vi "write error in txt.vi"(8 "error in (no error)":errorcluster caption="错误输入（无错误）", 9 "file name":string, 11 "path":path) -> (0 "error out":errorcluster, 3 "path":path)   [LabVIEW 2018]
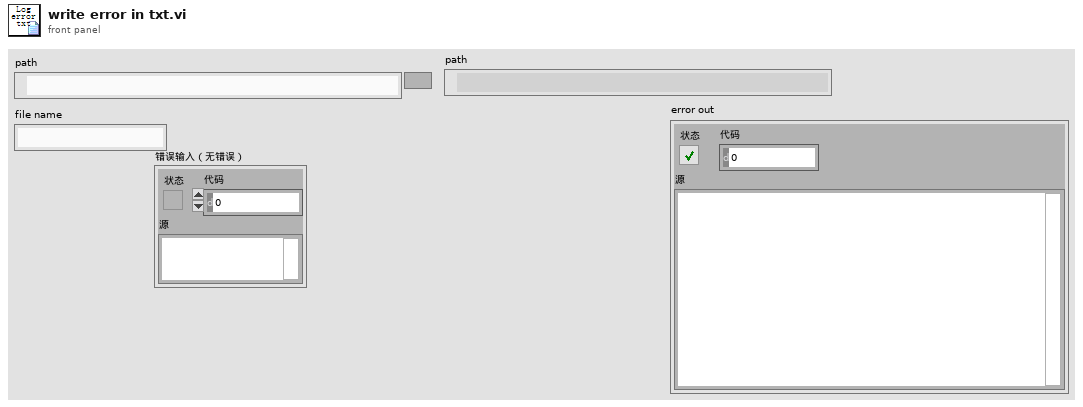
[diagram p1: front panel]
types:
  T1 = enum16{"open", "replace", "create", "open or create", "replace or create", "replace or create with confirmation"}
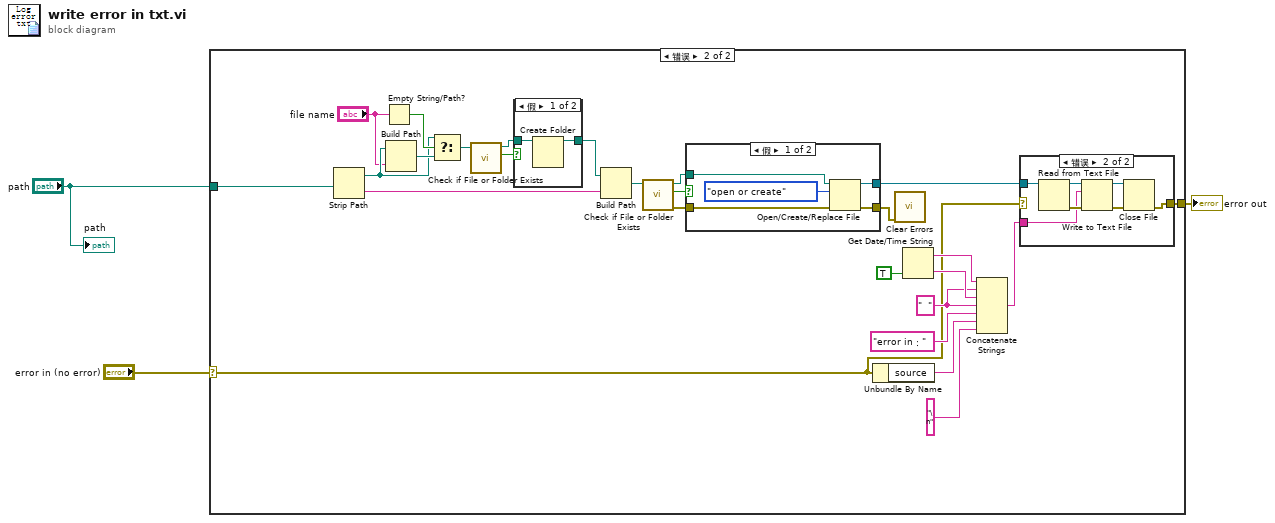
[diagram p0: block diagram]
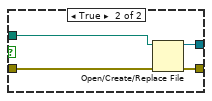
[diagram p5: hidden frame]
diagram:
  n1 = case shown="错误" "error in (no error)" {
    selector: "error in (no error)" -> [w4 w6]
    tunnel: [w4 w23] -> w3
    tunnel: "path" -> [_ w5]
    frame No Error {
    }
    frame Error {
      w27 = "  " ("字符串")
      n2 = Strip Path(path=w5) -> (stripped path=w10:path, name=w20:string)
      n3 = Empty String/Path?(string/path="file name") -> (empty?=w13:bool)
      n4 = Build Path(base path=w10, name or relative path="file name") -> (appended path=w11:path)
      n5 = Select(t=w10, s=w13, f=w11) -> (s? t:f=w12:path)
      n6 = call <vilib>:"Check if File or Folder Exists.vi"("path"=w12) -> ("file or folder exists?"=w15:bool, "dup path"=w14:path)  [unwired: 8 in, 1 out]
      n7 = case shown="假" w15 {
        tunnel: [w31 w33] -> w8
        tunnel: w14 -> [w32 w33]
        frame False {
          n8 = Create Folder(path (use dialog)=w32) -> (created path=w31:path)  [unwired: 2 in, 2 out]
        }
        frame True {
        }
      }
      n9 = Build Path(base path=w8, name or relative path=w20) -> (appended path=w18:path)
      n10 = call <vilib>:"Check if File or Folder Exists.vi"("path"=w18) -> ("error out"=w16:errorcluster, "file or folder exists?"=w17:bool, "dup path"=w19:path)  [unwired: 8 in]
      n11 = case shown="假" w17 {
        tunnel: [w44 w49] -> w22
        tunnel: w19 -> [w46 w50]
        tunnel: [w45 w48] -> w7
        tunnel: w16 -> [w42 w47]
        frame False {
          n12 = Open/Create/Replace File(file path (use dialog)=w46, error in=w42, operation (0:open)=T1."open or create" ("操作(0:open)")) -> (refnum out=w44:refnum<file>, error out=w45:errorcluster)  [unwired: 3 in, 1 out]
        }
        frame True {
          n13 = Open/Create/Replace File(file path (use dialog)=w50, error in=w47) -> (refnum out=w49:refnum<file>, error out=w48:errorcluster)  [unwired: 4 in, 1 out]
        }
      }
      n14 = Unbundle By Name(w6) -> ("source"=w25:string)
      n15 = call <vilib>:"Clear Errors.vi"("error in (no error)"=w7) -> ()  [unwired: 5 in, 2 out]
      n16 = Get Date/Time String(want seconds? (F)=TRUE ("需要秒？(F)")) -> (date string=w29:string, time string=w28:string)  [unwired: 2 in]
      n17 = Concatenate Strings(w29, w27, w28, w27, "error in：" ("字符串"), w25, "\n" ("字符串")) -> (w21:string)
      n18 = case shown="错误" w6 {
        selector: w6 -> [w34 _]
        tunnel: [w34 w39] -> w23
        tunnel: w22 -> [_ w38]
        tunnel: w21 -> [_ w35]
        frame No Error {
        }
        frame Error {
          n19 = Read from Text File(file (use dialog)=w38) -> (refnum out=w37:refnum<file>, error out=w36:errorcluster)  [unwired: 3 in, 2 out]
          n20 = Write to Text File(file (use dialog)=w37, text=w35, error in=w36) -> (refnum out=w41:refnum<file>, error out=w40:errorcluster)  [unwired: 1 in, 1 out]
          n21 = Close File(refnum=w41, error in=w40) -> (error out=w39:errorcluster)  [unwired: 1 out]
        }
      }
    }
  }
  "error out" <- w3
  "path" <- "path"
